vi "Validate Instrument Revision.vi"(0 "VISA resource name":refnum<visa-resource-name>, 11 "error in (no error)":errorcluster) -> (4 "VISA resource name out":refnum<visa-resource-name>, 6 "Firmware Version":string, 10 "Model Number":enum16{"6605", "6610", "6620", "6630", "6650"}(ring), 15 "error out":errorcluster)   [LabVIEW 2020, in "eec 6700.lvlib"]
doc: "Queries the instrument for the model number and firmware revision and validates them."
uses:
  <instrlib>/eec 6700/eec 6700.lvlib
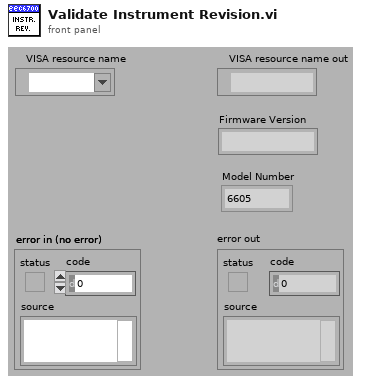
[diagram p1: front panel]
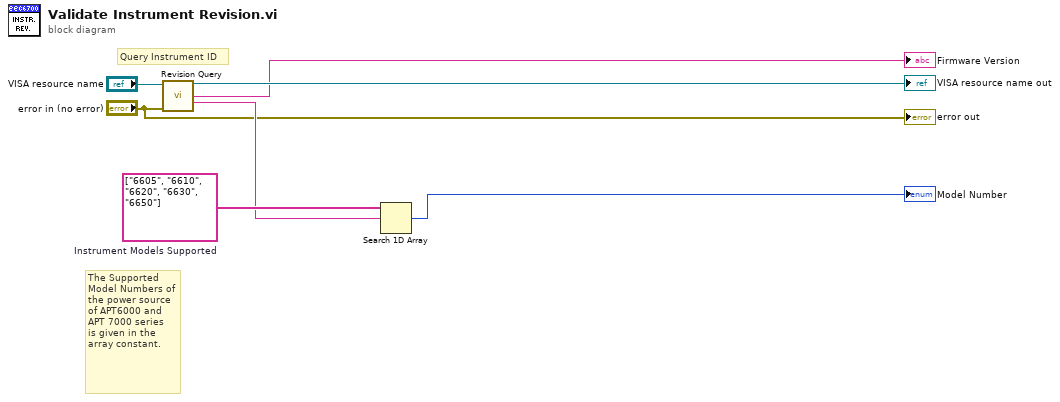
[diagram p0: block diagram]
diagram:
  w6 = string[] ["6605", "6610", "6620", "6630", "6650"]  # Instrument Models Supported
  # "The Supported Model Numbers of\nthe power source of APT6000 and APT 7000 series\nis given in the array constant."
  # "Query Instrument ID"
  n1 = call <instrlib>:"Revision Query.vi"("VISA resource name"="VISA resource name", "error in (no error)"="error in (no error)") -> ("VISA resource name out"=→"VISA resource name out":refnum<visa-resource-name>, "Instrument Firmware Revision"=→"Firmware Version":string, "Instrument Model"=w3:string)  [unwired: 9 in, 2 out]
  n2 = Search 1D Array(1D array=w6, element=w3) -> (index of element=→"Model Number":i32)  [unwired: 1 in]
  "error out" <- "error in (no error)"
